vi "SigToInfo.vi"(1 "Sig":string) -> (0 "Info":T1(array[cluster]))   [LabVIEW 2014]
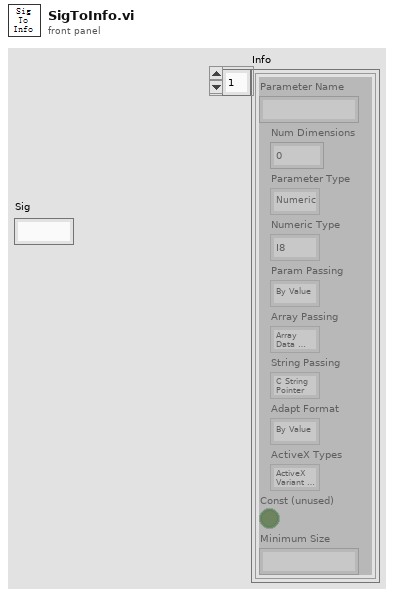
[diagram p1: front panel]
types:
  T1 = cluster{"Parameter Name":string, "Num Dimensions":i32, "Parameter Type":enum16{"Numeric", "Array", "String", "Waveform", "Digital Waveform", "Digital Table", "ActiveX", "Any", "Instance Data Pointer", "Void"}, "Numeric Type":enum16{"I8", "I16", "I32", "I64", "U8", "U16", "U32", "U64", "SGL", "DBL", "PTR INT", "PTR UINT"}, "Param Passing":enum16{"By Value", "Pointer To Value"}, "Array Passing":enum16{"Array Data Pointer", "Array Handle", "Array Handle Pointer"}, "String Passing":enum16{"C String Pointer", "Pascal String Pointer", "String Handle", "String Handle Pointer"}, "Adapt Format":enum16{"By Value", "Pointer To Value"}, "ActiveX Types":enum16{"ActiveX Variant Pointer", "IDispatch* Pointer", "IUnknown* Pointer"}, "Const (unused)":bool, "Minimum Size":string}[]
  T2 = cluster{"Parameter Name":string, "Num Dimensions":i32, "Parameter Type":enum16{"Numeric", "Array", "String", "Waveform", "Digital Waveform", "Digital Table", "ActiveX", "Any", "Instance Data Pointer", "Void"}, "Numeric Type":enum16{"I8", "I16", "I32", "I64", "U8", "U16", "U32", "U64", "SGL", "DBL", "PTR INT", "PTR UINT"}, "Param Passing":enum16{"By Value", "Pointer To Value"}, "Array Passing":enum16{"Array Data Pointer", "Array Handle", "Array Handle Pointer"}, "String Passing":enum16{"C String Pointer", "Pascal String Pointer", "String Handle", "String Handle Pointer"}, "Adapt Format":enum16{"By Value", "Pointer To Value"}, "ActiveX Types":enum16{"ActiveX Variant Pointer", "IDispatch* Pointer", "IUnknown* Pointer"}, "Const (unused)":bool, "Minimum Size":string}
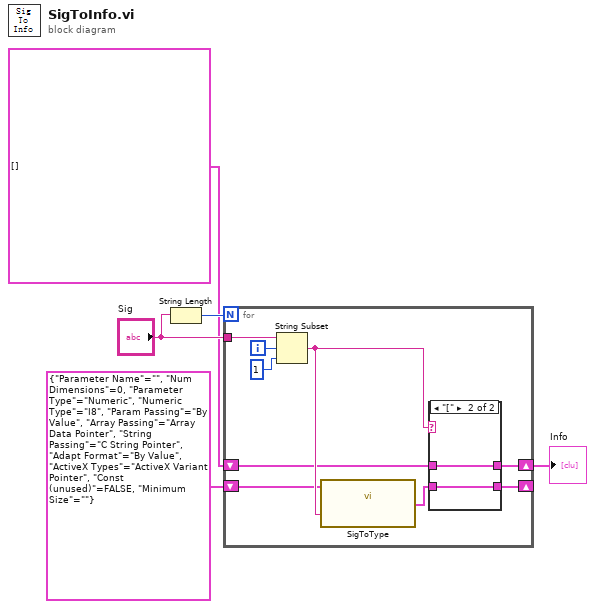
[diagram p0: block diagram]
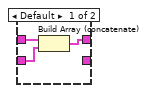
[diagram p2: hidden frame]
diagram:
  n1 = String Length(string="Sig") -> (length=w3:i32)
  n2 = for {
    N: w3 -> [_]
    tunnel: "Sig" -> [w14]
    shift-right: [w8] -> w5
    shift-left: T1 [] -> [w9]
    shift-right: [w7] -> _
    shift-left: T2 {"Parameter Name"="", "Num Dimensions"=0, "Parameter Type"=enum."Numeric", "Numeric Type"=enum."I8", "Param Passing"=enum."By Value", "Array Passing"=enum."Array Data Pointer", "String Passing"=enum."C String Pointer", "Adapt Format"=enum."By Value", "ActiveX Types"=enum."ActiveX Variant Pointer", "Const (unused)"=FALSE, "Minimum Size"=""} ("Output") -> [w6]
    i -> [w13]
    n3 = String Subset(string=w14, offset (0)=w13, length (rest)=1 ("length (rest)")) -> (substring=w11:string)
    n4 = call "SigToType.vi"("Sig"=w11, "Input"=w6) -> ("Output"=w10:T2)
    n5 = case shown="\"[\"" w11 {
      tunnel: w10 -> [w16 w18]
      tunnel: w9 -> [w17 w19]
      tunnel: [w15 w19] -> w8
      tunnel: [_ w18] -> w7
      frame Default {
        n6 = Build Array (concatenate)(w17, w16) -> (w15:T1)
      }
      frame "[" {
      }
    }
  }
  "Info" <- w5
